vi "DisableAllChannels.vi"(8 "error in (no error)":errorcluster, 11 "NISTFGenPluginsBase in":refnum<class "NISTFGenPluginsBase.lvclass">) -> (0 "error out":errorcluster, 3 "NISTFGenPluginsBase out":refnum<class "NISTFGenPluginsBase.lvclass">)   [LabVIEW 2014, in "FGenPlugins.lvlib" / "NISTFGenPluginsBase.lvclass"]
uses:
  NISTFGenPluginsBase.lvclass
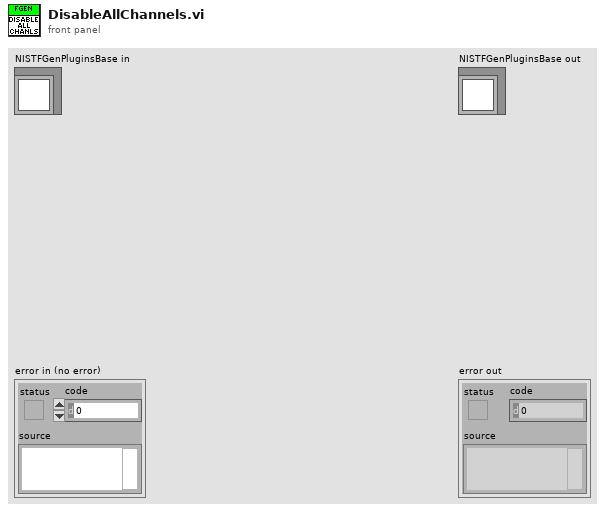
[diagram p1: front panel]
types:
  T1 = typedef "FGenPlugins.lvlib/NISTFGenPluginsBase.lvclass/ChannelParamElement.ctl" = cluster{"sName":string, "eOperateMode":u16, "bEnabled":bool, "eOutputMode":u16, "iIndex":i32, "iNameBufferSize":i32, "fGain":dbl}
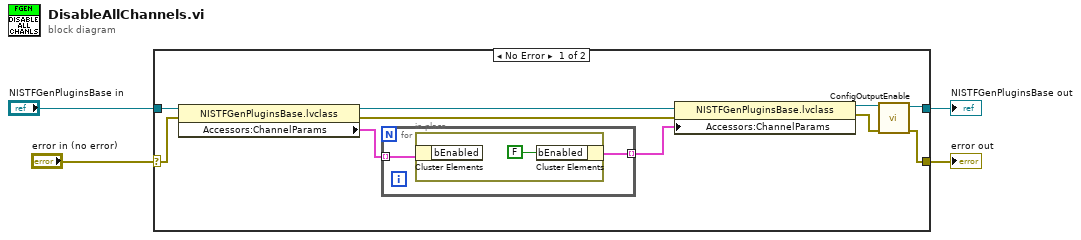
[diagram p0: block diagram]
diagram:
  n1 = case shown="No Error" "error in (no error)" {
    selector: "error in (no error)" -> [w11 w19]
    tunnel: [w5 w19] -> w3
    tunnel: [w7 w18] -> w1
    tunnel: "NISTFGenPluginsBase in" -> [w13 w18]
    frame No Error {
      n2 = property class="NISTFGenPluginsBase.lvclass"(reference=w13, error in=w11) -> (reference out=w12:refnum<class "NISTFGenPluginsBase.lvclass">, error out=w10:errorcluster, "Accessors:ChannelParams"=w14:T1[])
      n3 = for {
        tunnel: w14 -> [w16] mode=indexing
        tunnel: [w15] -> w9 mode=indexing
        n4 = in-place {
          n5 = in-place-cluster #1(w16) -> ()  [unwired: 1 out]
          n6 = in-place-cluster #1("bEnabled"=FALSE) -> (w15:T1)
        }
      }
      n7 = property class="NISTFGenPluginsBase.lvclass"(reference=w12, error in=w10, "Accessors:ChannelParams"=w9) -> (reference out=w8:refnum<class "NISTFGenPluginsBase.lvclass">, error out=w6:errorcluster)
      n8 = call-dynamic "ConfigOutputEnable.vi"("error in (no error)"=w6, "ClassIn"=w8) -> ("error out"=w5:errorcluster, "ClassOut"=w7:refnum<class "NISTFGenPluginsBase.lvclass">)  [unwired: 8 in]
    }
    frame Error {
    }
  }
  "error out" <- w3
  "NISTFGenPluginsBase out" <- w1
